vi "Enable EXFO Panel.vi"(8 "error in":errorcluster, 10 "Lock":bool, 11 "LTB-1 in":refnum<class "LTB-1.lvclass">) -> (0 "error out":errorcluster, 3 "LTB-1 out":refnum<class "LTB-1.lvclass">)   [LabVIEW 2018]
doc: "This is the parent method VI, the child class will use the appropriate calls to lock or unlock the front panel controls on the EXFO to prevent technicians inadvertently changing the configurtation.\n\nAuthor: Ron Dexter\nCompany: Luminar\nModified: 5/20/2018"
uses:
  LTB-1.lvclass
  C:/AME Test Engineering/LabVIEW/PPLs/EXFO/Parent/EXFO.lvlibp/EXFO.lvclass
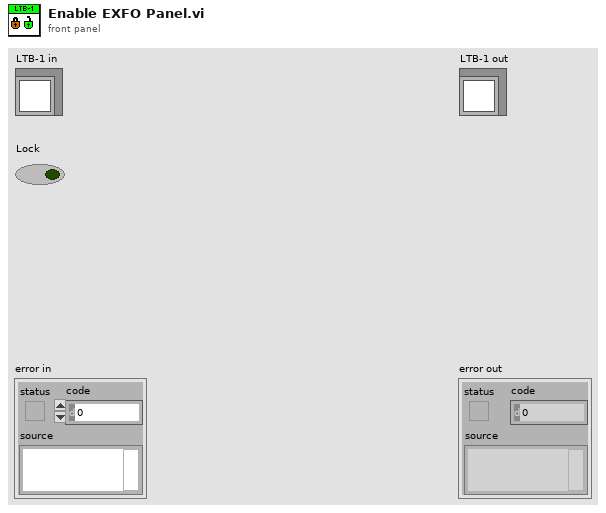
[diagram p1: front panel]
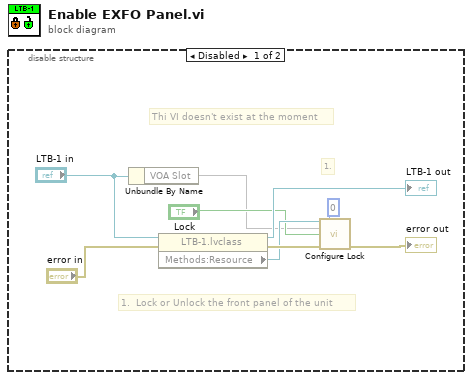
[diagram p0: block diagram]
diagram:
  n1 = disable-structure shown="Disabled" {
    frame Disabled {
      # "Thi VI doesn't exist at the moment"
      # "1.  Lock or Unlock the front panel of the unit"
      # "1."
      n2 = Unbundle By Name("LTB-1 in") -> ("VOA Slot"=w1)
      n3 = property class="LTB-1.lvclass"(reference="LTB-1 in", error in="error in") -> (reference out=→"LTB-1 out":refnum<class "LTB-1.lvclass">, error out=w5:errorcluster, "Methods:Resource"=w4:refnum<visa-resource-name>)
      n4 = call <instrlib>:"Configure Lock.vi"("VISA resource name"=w4, "Platform"=i16 0, "Module Slot Number (10)"=w1, "Lock Display (F:OFF)"="Lock", "error in (no error)"=w5) -> ("error out"=→"error out":errorcluster)  [unwired: 9 in, 1 out]
    }
    frame Enabled {
    }
  }
